vi "Value_to_string.vi"(1 "precision":string, 2 "Value":dbl=-999.0 format="%.5e", 3 "Label for value":string) -> (0 "Output string":string)   [LabVIEW 2010]
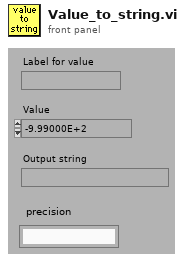
[diagram p1: front panel]
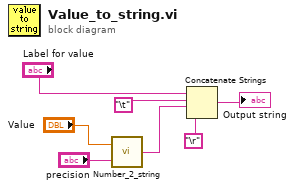
[diagram p0: block diagram]
diagram:
  n1 = call "Number_2_string.vi"("precision"="precision", "number"="Value") -> ("String"=w2:string)
  n2 = Concatenate Strings("Label for value", "\t", w2, "\r") -> (→"Output string":string)
